vi "1-6 Demux.vi"(0 "input":bool, 6 "select":u8) -> (14 "output 0":bool, 15 "output 1":bool, 16 "output 2":bool, 17 "output 3":bool, 18 "output 4":bool, 19 "output 5":bool)   [LabVIEW 2016]
doc: "Sets the <B>output</B> to the <B>input</B> that you specify in the <B>select</B> parameter."
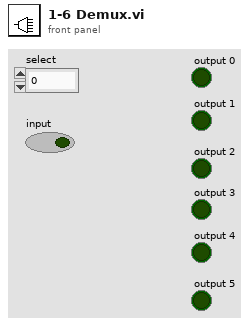
[diagram p1: front panel]
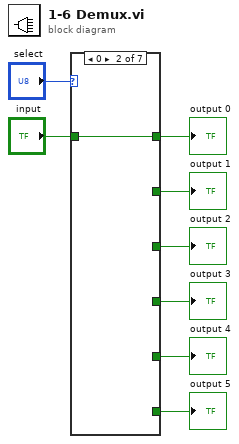
[diagram p0: block diagram]
diagram:
  n1 = case shown="0" "select" {
    tunnel: "input" -> [_ w9 w10 w11 w12 w13 w14]
    tunnel: [_ w9 _ _ _ _ _] -> w7
    tunnel: [_ _ w10 _ _ _ _] -> w5
    tunnel: [_ _ _ w11 _ _ _] -> w4
    tunnel: [_ _ _ _ w12 _ _] -> w3
    tunnel: [_ _ _ _ _ w13 _] -> w2
    tunnel: [_ _ _ _ _ _ w14] -> w1
    frame Default {
    }
    frame 0 {
    }
    frame 1 {
    }
    frame 2 {
    }
    frame 3 {
    }
    frame 4 {
    }
    frame 5 {
    }
  }
  "output 0" <- w7
  "output 1" <- w5
  "output 2" <- w4
  "output 5" <- w1
  "output 3" <- w3
  "output 4" <- w2
